vi "Lab 9 Exercise 8 - State Machine.vi"() -> ()   [LabVIEW 2023]
doc: "Use this template to build a simple state machine design pattern. Each state executes code and determines which state to transition to."
uses:
  Documents/LabVIEW Data/Lab 9 Exercise 8/controls/State.ctl
panel:
  out "Current State":T1
  # "These controls have associated \"Value Changed\" events configured in the Event Structure on the diagram.\n\nReplace them (and reconfigure the Event Structure) with the controls you need for your application."
  # "This template is for the Simple State Machine design pattern.\n\nSee the block diagram for more information on how to use this template."
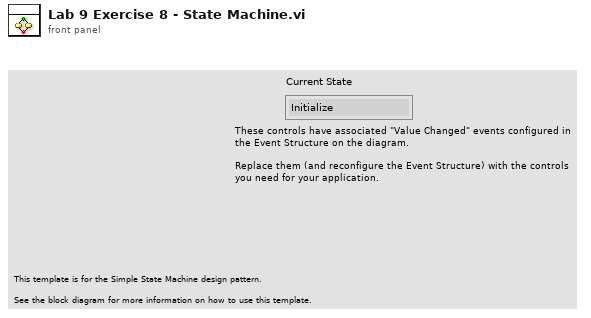
[diagram p1: front panel]
types:
  T1 = typedef "State.ctl" = enum16{"Initialize", "Stop", "State 1", "State 2"}
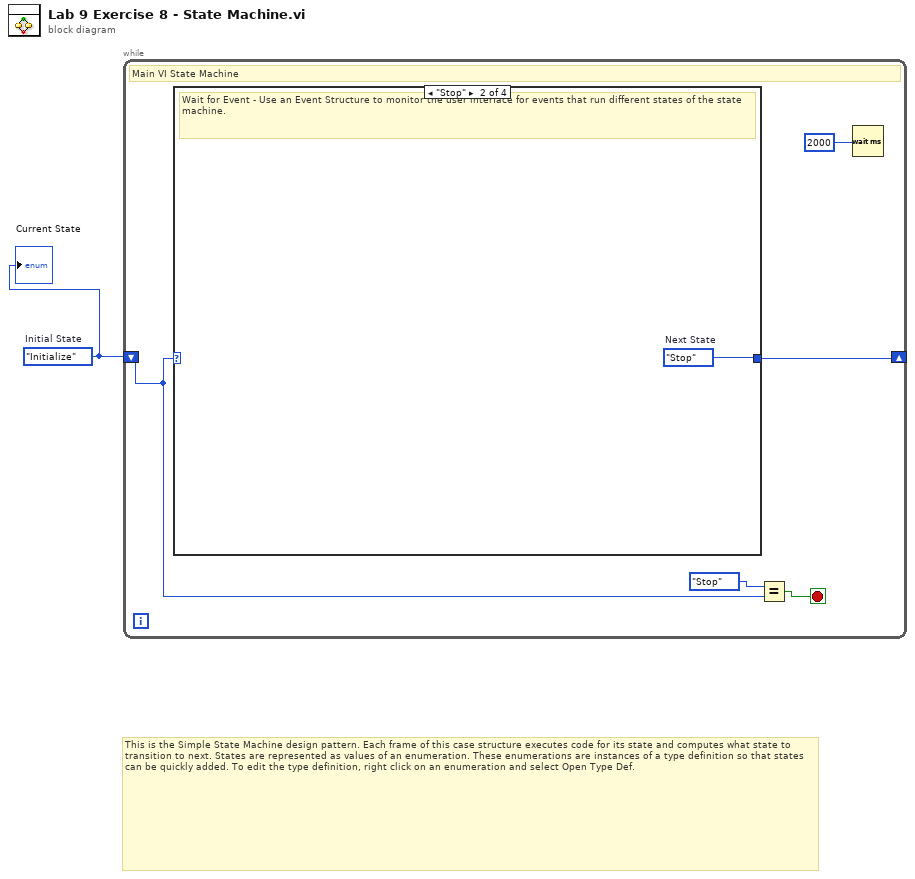
[diagram p0: block diagram]
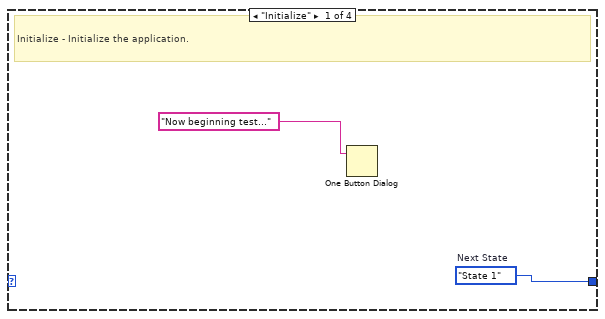
[diagram p2: hidden frame]
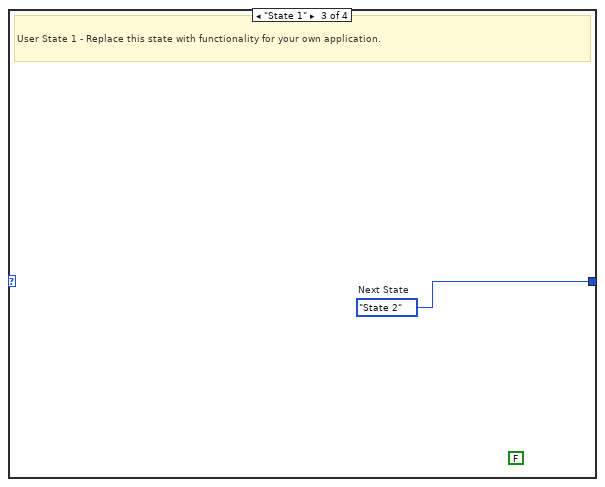
[diagram p3: hidden frame]
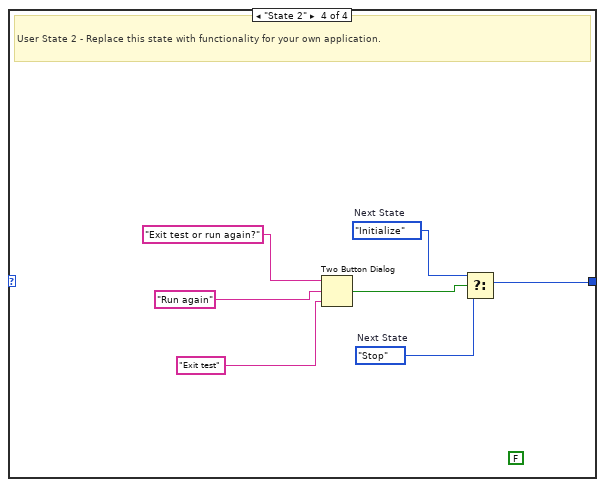
[diagram p4: hidden frame]
diagram:
  w1 = State."Initialize"  # Initial State
  # "This is the Simple State Machine design pattern. Each frame of this case structure executes code for its state and computes what state to transition to next. States are represented as values of an enumeration. These enumerations are instances of a type definition so that states can be quickly added. To edit the type definition, right click on an enumeration and select Open Type Def."
  n1 = while {
    shift-right: [w5] -> _
    shift-left: w1 -> [w4]
    stop <- w3 stop-if-true
    # "Main VI State Machine"
    n2 = case shown="\"Stop\"" w4 {
      tunnel: [w7 w9 w10 w16] -> w5
      frame "Initialize" {
        w7 = State."State 1"  # Next State
        # "Initialize - Initialize the application."
        n3 = One Button Dialog(message="Now beginning test...") -> ()  [unwired: 1 in, 1 out]
      }
      frame "Stop" {
        w9 = State."Stop"  # Next State
        # "Wait for Event - Use an Event Structure to monitor the user interface for events that run different states of the state machine."
      }
      frame "State 1" {
        w10 = State."State 2"  # Next State
        (unwired) FALSE ("Stop Loop?")
        # "User State 1 - Replace this state with functionality for your own application."
      }
      frame "State 2" {
        w15 = State."Initialize"  # Next State
        w17 = State."Stop"  # Next State
        (unwired) FALSE ("Stop Loop?")
        # "User State 2 - Replace this state with functionality for your own application."
        n4 = Two Button Dialog(message="Exit test or run again?", 1:"Exit test", 2:"Run again") -> (T button?=w14:bool)
        n5 = Select(t=w15, s=w14, f=w17) -> (s? t:f=w16:T1)
      }
    }
    n6 = Equal?(x=State."Stop", y=w4) -> (x = y?=w3:bool)
    n7 = Wait (ms)(milliseconds to wait=2000) -> ()  [unwired: 1 out]
  }
  "Current State" <- w1
